vi "BRig_generic_convert__Prob_to_TrueFalse__numeric.vi"(11 "input_probability_u16":u16) -> (3 "output_TF":u16)   [LabVIEW 2014]
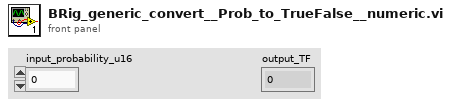
[diagram p1: front panel]
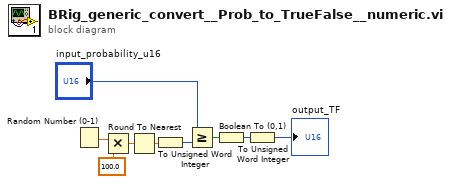
[diagram p0: block diagram]
diagram:
  n1 = Random Number (0-1)() -> (number: 0 to 1=w9:dbl)
  n2 = Multiply(x=w9, y=100.0) -> (x*y=w8:dbl)
  n3 = Round To Nearest(number=w8) -> (nearest integer value=w7:dbl)
  n4 = To Unsigned Word Integer(number=w7) -> (unsigned 16bit integer=w6:u16)
  n5 = Greater Or Equal?(x="input_probability_u16", y=w6) -> (x >= y?=w3:bool)
  n6 = Boolean To (0,1)(Boolean=w3) -> (0, 1=w2:i16)
  n7 = To Unsigned Word Integer(number=w2) -> (unsigned 16bit integer=→"output_TF":u16)
